vi "Main Interface.vi"() -> ()   [LabVIEW 2015]
uses:
  Ctrls/Data operation control.ctl
  <vilib>/Utility/error.llb/DialogType.ctl
  <vilib>/DAQmx/read.llb/DAQmx Read (Counter U32 1Chan 1Samp).vi
  <vilib>/DAQmx/create/channels.llb/DAQmx Create Channel (CI-Count Edges).vi
  <vilib>/DAQmx/miscellaneous.llb/DAQmx Fill In Error Info.vi
  <resource>/objmgr/daqmx.rc
panel:
  in  "Row add 1":bool
  in  "Enum":enum16{"Zero", "Full code", "No compare"}(ring)
  in  "Tab Control":enum32{"Parameter Setup", "Map", "Data"}(tab)
  in  "Timelapse per pixel (ms)":i32=100
  in  "Size of a single pixel (um)":dbl=0.018
  in  "Quantity of Pixels of one step":dbl=6.0
  in  "X direction total length- Width (um)":dbl=1.15
  in  "Y direction total length- Height (um)":dbl=1.66
  in  "counter":tag="Dev3/ctr2"
  in  "CI.CountEdges.Term":tag="/Dev3/PFI0"
  out "SEE Scanning Map":dbl[][](graph)
  out "Number of Rows":i32
  out "Number of Volumns":i32
  out "Length of each step":dbl
  out "Galvo":bool
  in  "Reset":bool
  in  "stop":bool
  out "Total steps":i32
  in  "Current Step":i32
  out "output array":dbl[][](array[numeric])
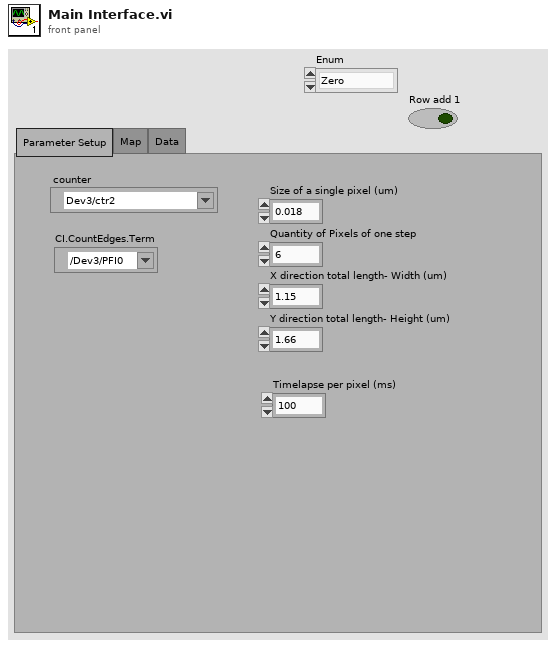
[diagram p1: front panel]
types:
  T1 = typedef "DialogType.ctl" = u16
  T2 = typedef "Data operation control.ctl" = cluster{"States":enum16{"Initializtion", "SEE maping", "Exit"}, "SEE data":i32}
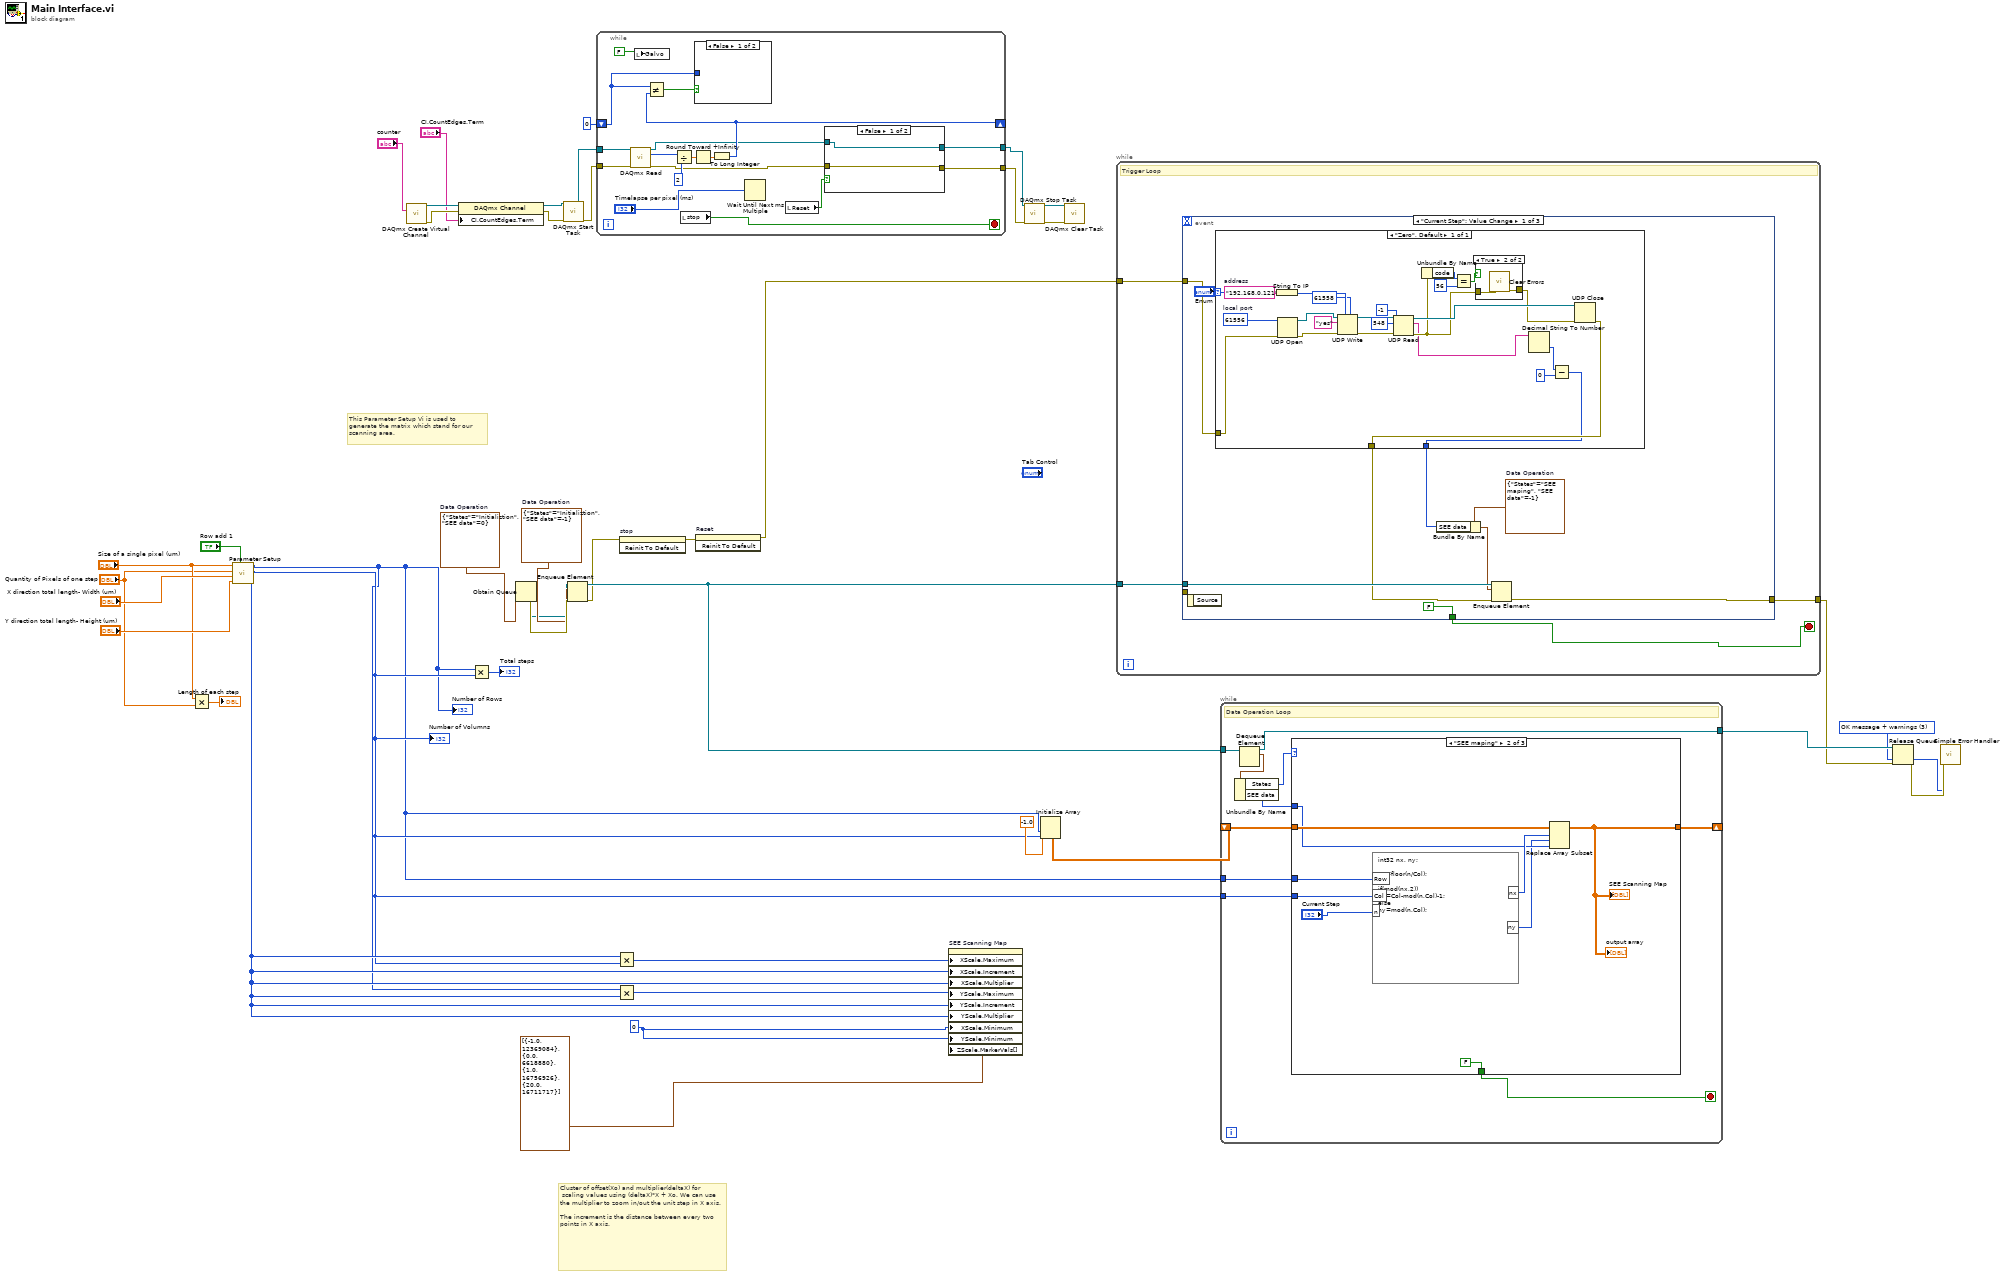
[diagram p0: block diagram]
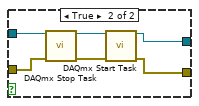
[diagram p2: hidden frame]
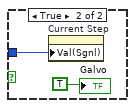
[diagram p3: hidden frame]
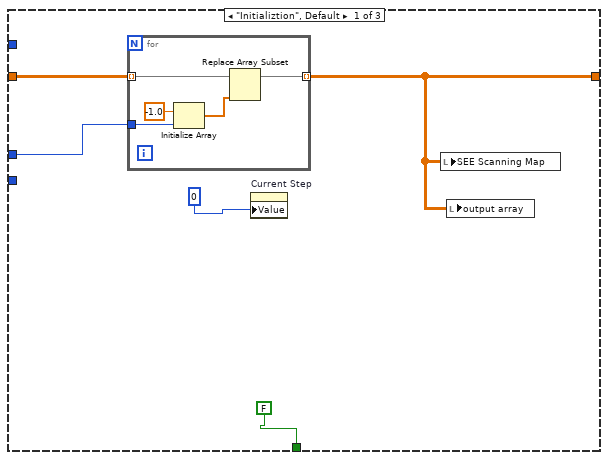
[diagram p4: hidden frame]
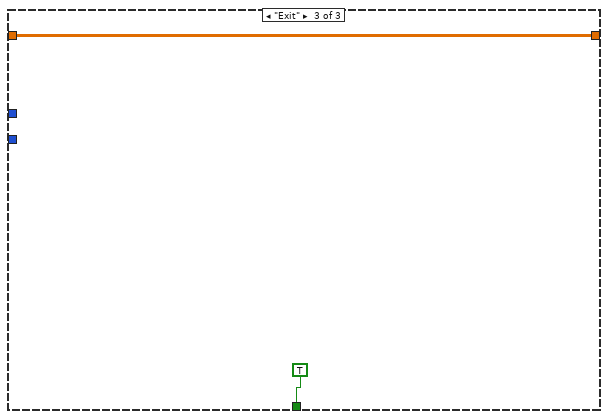
[diagram p5: hidden frame]
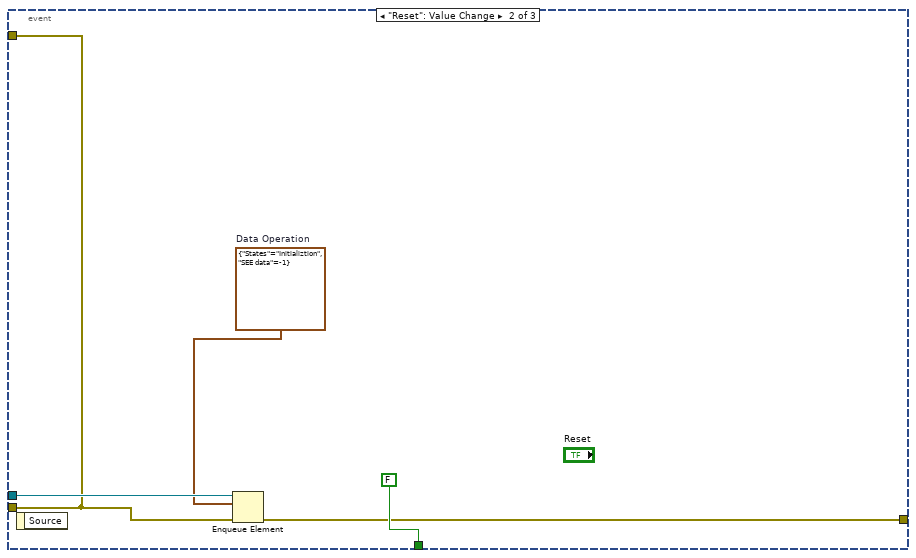
[diagram p7: hidden frame]
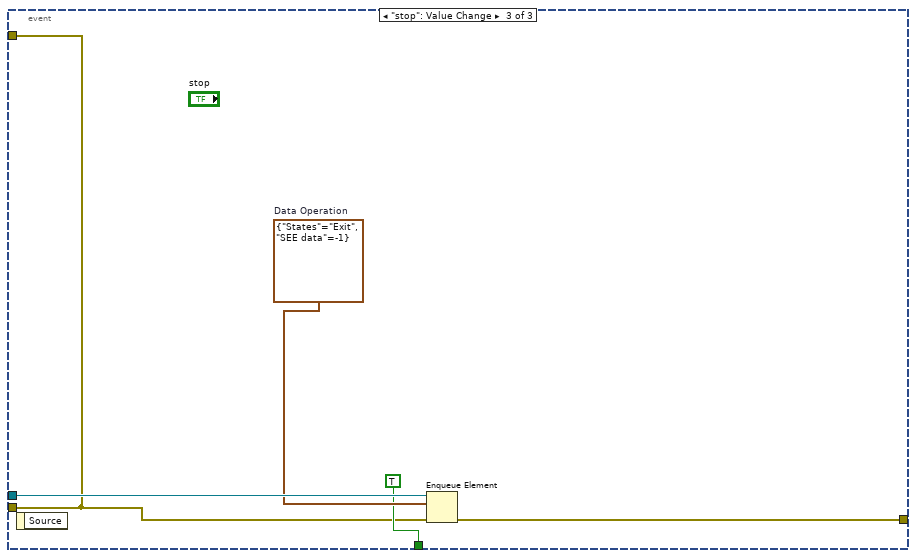
[diagram p8: hidden frame]
diagram:
  w25 = T1 3 items=["no dialog", "OK message", "continue or stop message", "OK message + warnings", "continue/stop + warnings"] ("type of dialog (OK msg:1)")
  w28 = 0
  w37 = T2 {"States"=enum."Initializtion", "SEE data"=-1}  # Data Operation
  w39 = T2 {"States"=enum."Initializtion", "SEE data"=0}  # Data Operation
  # "This Parameter Setup Vi is used to \ngenerate the matrix which stand for our\nscanning area."
  # "Cluster of offset(Xo) and multiplier(deltaX) for\n scaling values using (deltaX)*X + Xo. We can use the multiplier to zoom in/out the unit step in X axis.\n\nThe increment is the distance between every two points in X axis."
  n1 = Multiply(x="Size of a single pixel (um)", y="Quantity of Pixels of one step") -> (x*y=→"Length of each step":dbl)
  n2 = call "Parameter Setup.vi"("Row add 1"="Row add 1", "Y direction total length- Height (um)"="Y direction total length- Height (um)", "X direction total length- Width (um)"="X direction total length- Width (um)", "Quantity of Pixels of one step"="Quantity of Pixels of one step", "Size of a single pixel (um)"="Size of a single pixel (um)") -> ("Length of each Step (um)"=w29:i32, "Number of Volumns"=w3:i32, "Number of Rows"=w2:i32)  [unwired: 4 in]
  "Number of Rows" <- w2
  "Number of Volumns" <- w3
  n3 = call-poly <vilib>:"DAQmx Create Virtual Channel.vi"("counter"="counter") -> ("task out"=w20:refnum<k21>, "error out"=w19:errorcluster)  [unwired: 13 in]
  n4 = property class="DAQmx Channel"(reference=w20, error in=w19, "CI.CountEdges.Term"="CI.CountEdges.Term") -> (reference out=w16:refnum<k21>, error out=w15:errorcluster)
  n5 = Multiply(x=w2, y=w3) -> (x*y=→"Total steps":i32)
  n6 = Obtain Queue(element data type=w39) -> (queue out=w36:refnum<queue>, error out=w38:errorcluster)  [unwired: 4 in, 1 out]
  n7 = call <vilib>:"DAQmx Start Task.vi"("task/channels in"=w16, "error in"=w15) -> ("task out"=w14:refnum<k21>, "error out"=w13:errorcluster)  [unwired: 12 in]
  n8 = Enqueue Element(queue=w36, element=w37, error in (no error)=w38) -> (queue out=w35:refnum<queue>, error out=w7:errorcluster)  [unwired: 1 in, 1 out]
  n9 = while {
    tunnel: w14 -> [w58]
    tunnel: w13 -> [w57]
    shift-right: [w48] -> _
    shift-left: u32 0 ("data") -> [w52]
    tunnel: [w42] -> w11
    tunnel: [w44] -> w9
    stop <- w53 stop-if-true
    n10 = call-poly <vilib>:"DAQmx Read.vi"("task/channels in"=w58, "error in"=w57) -> ("task out"=w46:refnum<k21>, "data"=w56:u32, "error out"=w43:errorcluster)  [unwired: 11 in]
    n11 = local write "Galvo"(FALSE) -> ()
    n12 = Divide(x=w56, y=u32 2) -> (x/y=w50:dbl)
    n13 = local read "stop"() -> (w53:bool)
    n14 = Round Toward +Infinity(x=w50) -> (ceil(x): smallest int >= x=w49:dbl)
    n15 = To Long Integer(number=w49) -> (32bit integer=w48:i32)
    n16 = Not Equal?(x=w52, y=w48) -> (x != y?=w54:bool)
    n17 = case shown="False" w54 {
      tunnel: w52 -> [_ w68]
      frame False {
      }
      frame True {
        n18 = property on="Current Step" class="DigNum (strict)"("Val(Sgnl)"=w68) -> ()  [unwired: 2 in, 2 out]
        "Galvo" <- TRUE
      }
    }
    n19 = Wait Until Next ms Multiple(millisecond multiple="Timelapse per pixel (ms)") -> ()  [unwired: 1 out]
    n20 = local read "Reset"() -> (w45:bool)
    n21 = case shown="False" w45 {
      tunnel: w46 -> [w60 w65]
      tunnel: [w60 w62] -> w44
      tunnel: w43 -> [w59 w66]
      tunnel: [w59 w61] -> w42
      frame False {
      }
      frame True {
        n22 = call <vilib>:"DAQmx Stop Task.vi"("task/channels in"=w65, "error in"=w66) -> ("task out"=w64:refnum<k21>, "error out"=w63:errorcluster)  [unwired: 12 in]
        n23 = call <vilib>:"DAQmx Start Task.vi"("task/channels in"=w64, "error in"=w63) -> ("task out"=w62:refnum<k21>, "error out"=w61:errorcluster)  [unwired: 12 in]
      }
    }
  }
  n24 = Multiply(x=w29, y=w3) -> (x*y=w31:i32)
  n25 = Multiply(x=w2, y=w29) -> (x*y=w30:i32)
  n26 = invoke on="stop" class="Bool (strict)" method="Reinit To Default"(error in=w7) -> (error out=w6:errorcluster)  [unwired: 2 in, 2 out]
  n27 = invoke on="Reset" class="Bool (strict)" method="Reinit To Default"(error in=w6) -> (error out=w5:errorcluster)  [unwired: 2 in, 2 out]
  n28 = property on="SEE Scanning Map" class="IntGraph (strict)"("XScale.Maximum"=w31, "XScale.Increment"=w29, "XScale.Multiplier"=w29, "YScale.Maximum"=w30, "YScale.Increment"=w29, "YScale.Multiplier"=w29, "XScale.Minimum"=w28, "YScale.Minimum"=w28, "ZScale.MarkerVals[]"=cluster{dbl, u32}[] [{-1.0, 12369084}, {0.0, 6618880}, {1.0, 16756926}, {20.0, 16711717}] ("Z Scale.Marker Values[]")) -> ()  [unwired: 2 in, 2 out]
  n29 = call <vilib>:"DAQmx Stop Task.vi"("task/channels in"=w9, "error in"=w11) -> ("task out"=w8:refnum<k21>, "error out"=w10:errorcluster)  [unwired: 12 in]
  n30 = Initialize Array(-1.0 ("element"), w2, w3) -> (w32:dbl[][])
  n31 = call <vilib>:"DAQmx Clear Task.vi"("task in"=w8, "error in"=w10) -> ()  [unwired: 13 in, 1 out]
  n32 = while {
    tunnel: w35 -> [w72]
    tunnel: [w71] -> w4
    tunnel: w5 -> [w69]
    stop <- w70 stop-if-true
    # "Trigger Loop"
    n33 = event shown="[0] \"Current Step\": Value Change" {
      selector: _ -> [_ _ _]
      dyn-events: _ -> [_ _ _]
      timeout: _ -> [_ _ _]
      tunnel: [FALSE FALSE TRUE] -> w70
      tunnel: w72 -> [w80 w112 w117]
      tunnel: [w79 w109 w116] -> w71
      tunnel: [_ w108 w113] -> _
      tunnel: w69 -> [w76 w108 w113]
      event "Current Step": Value Change {
        w78 = T2 {"States"=enum."SEE maping", "SEE data"=-1}  # Data Operation
        n34 = event-data() -> ()  [unwired: 1 in, 1 out]
        n35 = case shown="\"Zero\", Default" "Enum" {
          tunnel: w76 -> [w98]
          tunnel: [w92] -> w75
          tunnel: [w84] -> w74
          frame "Zero", Default {
            w103 = u16 61556  # local port
            w104 = "192.168.0.121"  # address
            n36 = String To IP(1:w104) -> (0:w102:u32)
            n37 = UDP Open(8:w98, 11:w103) -> (port=w100:refnum<k16>, 0:w97:errorcluster)  [unwired: 3 in, 1 out]
            n38 = UDP Write(address=w102, port or service name=u16 61558, connection ID=w100, data in="yes", 8:w97) -> (error out=w95:errorcluster, 3:w96:refnum<k16>)  [unwired: 1 in]
            n39 = UDP Read(connection ID=w96, max size (548)=548, timeout ms (25000)=-1, 8:w95) -> (data out=w83:string, error out=w88:errorcluster, 3:w93:refnum<k16>)  [unwired: 2 out]
            n40 = Unbundle By Name(w88) -> ("code"=w90:i32)
            n41 = Equal?(x=w90, y=56) -> (x = y?=w91:bool)
            n42 = case shown="True" w91 {
              tunnel: w88 -> [w105 w107]
              tunnel: [w105 w106] -> w87
              frame False {
              }
              frame True {
                n43 = call <vilib>:"Clear Errors.vi"("error in (no error)"=w107) -> ("error out"=w106:errorcluster)  [unwired: 5 in, 1 out]
              }
            }
            n44 = Decimal String To Number(string=w83) -> (number=w86:i32)  [unwired: 2 in, 1 out]
            n45 = Subtract(x=w86, y=0) -> (x-y=w84:i32)
            n46 = UDP Close(connection ID=w93, 8:w87) -> (error out=w92:errorcluster)  [unwired: 1 out]
          }
        }
        n47 = Bundle By Name(cluster=w78, "SEE data"=w74) -> (w77:T2)
        n48 = Enqueue Element(queue=w80, element=w77, error in (no error)=w75) -> (error out=w79:errorcluster)  [unwired: 1 in, 2 out]
      }
      event "Reset": Value Change {
        w111 = T2 {"States"=enum."Initializtion", "SEE data"=-1}  # Data Operation
        n49 = event-data() -> ()  [unwired: 1 in, 1 out]
        n50 = Enqueue Element(queue=w112, element=w111, error in (no error)=w108) -> (error out=w109:errorcluster)  [unwired: 1 in, 2 out]
      }
      event "stop": Value Change {
        w115 = T2 {"States"=enum."Exit", "SEE data"=-1}  # Data Operation
        n51 = event-data() -> ()  [unwired: 1 in, 1 out]
        n52 = Enqueue Element(queue=w117, element=w115, error in (no error)=w113) -> (error out=w116:errorcluster)  [unwired: 1 in, 2 out]
      }
    }
  }
  n53 = while {
    tunnel: w35 -> [w127]
    tunnel: [w124] -> w34
    shift-right: [w122] -> _
    shift-left: w32 -> [w123]
    tunnel: w2 -> [w120]
    tunnel: w3 -> [w119]
    stop <- w118 stop-if-true
    # "Data Operation Loop"
    n54 = Dequeue Element(queue=w127) -> (queue out=w124:refnum<queue>, element=w126:T2)  [unwired: 2 in, 2 out]
    n55 = Unbundle By Name(w126) -> ("States"=w125:enum16{"Initializtion", "SEE maping", "Exit"}, "SEE data"=w121:i32)
    n56 = case shown="\"SEE maping\"" w125 {
      tunnel: w123 -> [w131 w143 w148]
      tunnel: [w128 w140 w148] -> w122
      tunnel: w121 -> [_ w141 _]
      tunnel: w120 -> [w132 w145 _]
      tunnel: [FALSE FALSE TRUE] -> w118
      tunnel: w119 -> [_ w144 _]
      frame "Initializtion", Default {
        n57 = for {
          tunnel: w132 -> [w136]
          tunnel: w131 -> [w135] mode=indexing
          tunnel: [w134] -> w128 mode=indexing
          n58 = Initialize Array(-1.0 ("element"), w136) -> (w133:dbl[])
          n59 = Replace Array Subset(array=w135, new element=w133) -> (w134:dbl[])  [unwired: 1 in]
        }
        n60 = property on="Current Step" class="DigNum (strict)"("Value"=u32 0 ("Count")) -> ()  [unwired: 2 in, 2 out]
        n61 = local write "SEE Scanning Map"(w128) -> ()
        n62 = local write "output array"(w128) -> ()
      }
      frame "SEE maping" {
        n63 = formula code="int32 nx, ny;\n\nnx=floor(n/Col); \n\nif(mod(nx,2))\nny=Col-mod(n,Col)-1; \nelse\nny=mod(n,Col);"("Row"=w145, "Col"=w144, "n"="Current Step") -> ("nx"=w142:i32, "ny"=w139:i32)
        n64 = Replace Array Subset(array=w143, new element=w141, index (row)=w142, index (col)=w139) -> (w140:dbl[][])
        "SEE Scanning Map" <- w140
        "output array" <- w140
      }
      frame "Exit" {
      }
    }
  }
  n65 = Release Queue(queue=w34, error in (no error)=w4) -> (error out=w26:errorcluster)  [unwired: 1 in, 2 out]
  n66 = call <vilib>:"Simple Error Handler.vi"("type of dialog (OK msg:1)"=w25, "error in (no error)"=w26) -> ()  [unwired: 3 in, 5 out]
